vi "Make Leaf Outcome Rectangles.vi"(7 "Leaf Circle Radius":dbl, 9 "Height Padding":dbl, 10 "Width Padding":dbl, 11 "Drawing Info in":T1) -> (0 "Leaf Circle Center":cluster{"mean":dbl, dbl}, 3 "Text Rectangle":T1)   [LabVIEW 2025]
uses:
  <vilib>/Analysis/baseanly.llb/Mean (DBL).vi
  <vilib>/Analysis/NI_AALBase.lvlib
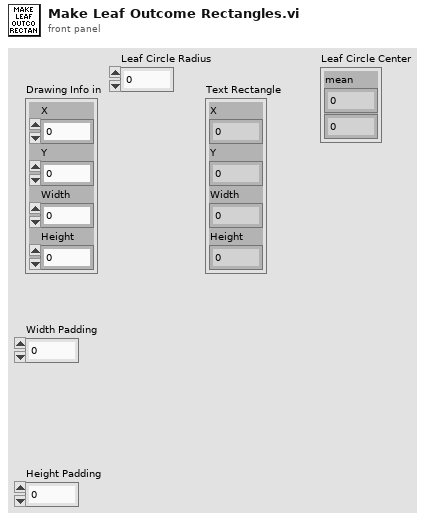
[diagram p1: front panel]
types:
  T1 = cluster{"X":dbl, "Y":dbl, "Width":dbl, "Height":dbl}
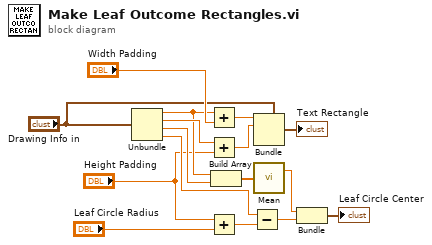
[diagram p0: block diagram]
diagram:
  n1 = Unbundle("Drawing Info in") -> ("X"=w9:dbl, "Y"=w16:dbl, "Width"=w8:dbl, "Height"=w10:dbl)
  n2 = Add(x=w9, y="Width Padding") -> (x+y=w14:dbl)
  n3 = Add(x=w16, y="Height Padding") -> (x+y=w12:dbl)
  n4 = Add(x="Height Padding", y="Leaf Circle Radius") -> (x+y=w4:dbl)
  n5 = Build Array(w9, w8) -> (w7:dbl[])
  n6 = Subtract(x=w10, y=w4) -> (x-y=w2:dbl)
  n7 = Bundle(cluster="Drawing Info in", "X"=w14, "Y"=w12) -> (→"Text Rectangle":T1)  [unwired: 2 in]
  n8 = call-poly <vilib>:"Mean.vi"("X"=w7) -> ("mean"=w3:dbl)  [unwired: 1 out]
  n9 = Bundle("mean"=w3, w2) -> (→"Leaf Circle Center":cluster{"mean":dbl, dbl})  [unwired: 1 in]
